vi "run_vi.vi"(6 "wait for reply (T)":bool=TRUE, 8 "error in":errorcluster, 9 "open_frontpanel":bool, 10 "vi_id":i32) -> (0 "error out":errorcluster, 1 "timed out?":bool)   [LabVIEW 2025, in "Scripting Server.lvlib"]
doc: "Runs a VI specified by VI ID and brings the frontpanel to foreground if open_frontpanel is set to True."
uses:
  Scripting Server.lvlib
  Run VI Argument--cluster.ctl
  Run VI (Reply Payload)--cluster.ctl
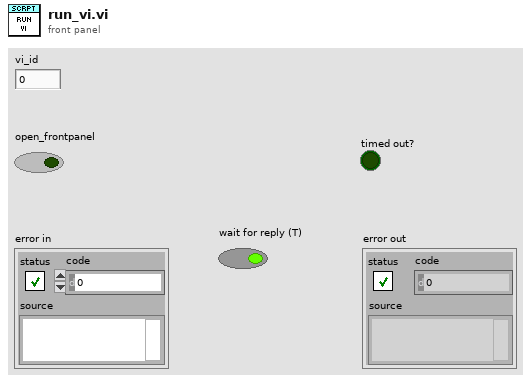
[diagram p1: front panel]
types:
  T1 = typedef "Scripting Server.lvlib/Run VI Argument--cluster.ctl" = cluster{"VI ID":i32, "open_frontpanel":bool, "Wait Notifier":refnum<notifier>, "wait for reply":bool}
  T2 = typedef "Scripting Server.lvlib/Request Events--cluster.ctl" = cluster{"Stop Module":refnum<user-event>, "Show Panel":refnum<user-event>, "Hide Panel":refnum<user-event>, "Get Module Execution Status":refnum<user-event>, "Show Diagram":refnum<user-event>, "New VI":refnum<user-event>, "Add Object":refnum<user-event>, "Connect Objects":refnum<user-event>, "Get Object Terminals":refnum<user-event>, "get vi error list":refnum<user-event>, "Cleanup VI":refnum<user-event>, "create_control":refnum<user-event>, "Run VI":refnum<user-event>}
  T3 = typedef "Scripting Server.lvlib/Run VI (Reply Payload)--cluster.ctl" = cluster{"error":errorcluster}
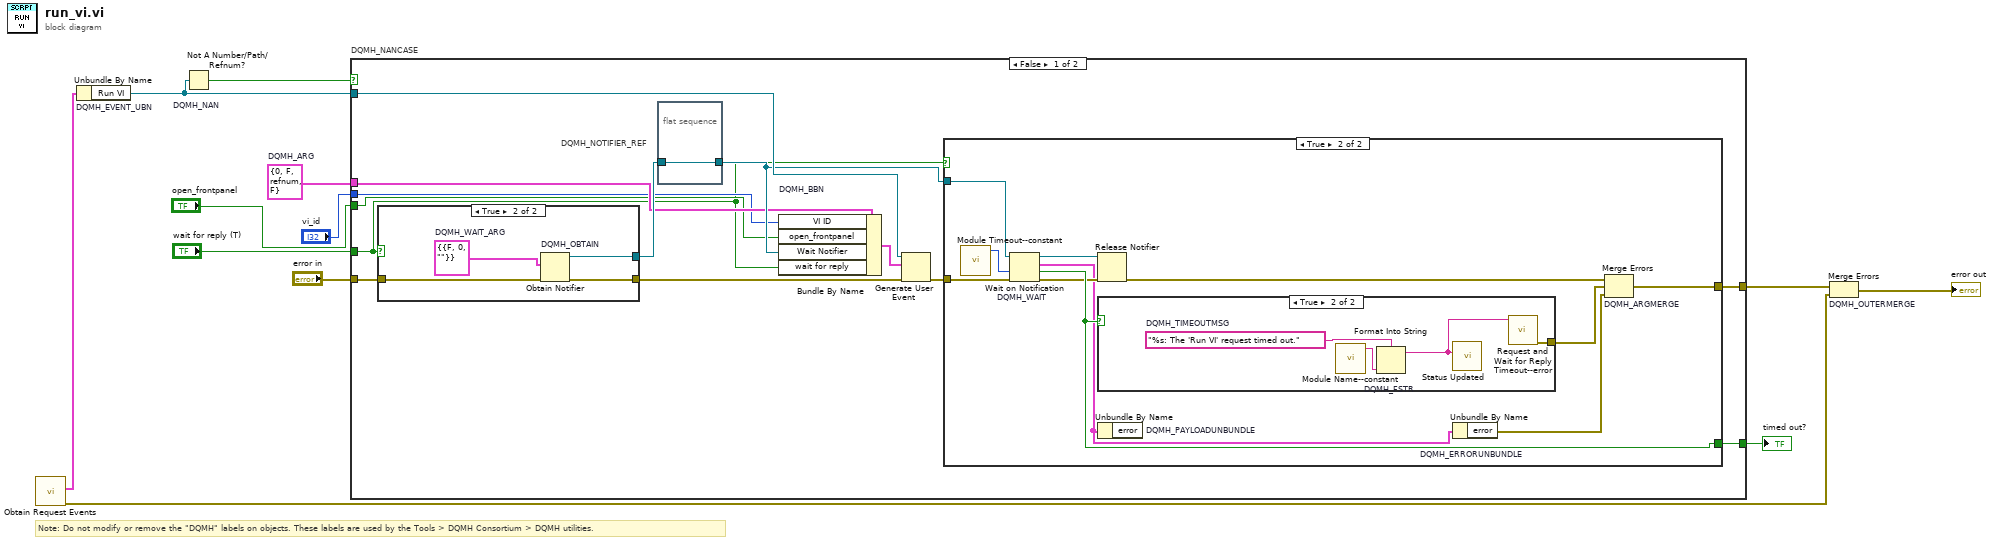
[diagram p0: block diagram]
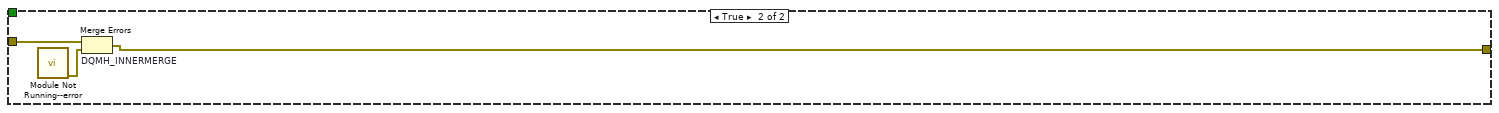
[diagram p5: hidden frame]
diagram:
  w6 = T1 {"VI ID"=0, "open_frontpanel"=FALSE, "Wait Notifier"=refnum, "wait for reply"=FALSE}  # DQMH_ARG
  # "Note: Do not modify or remove the \"DQMH\" labels on objects. These labels are used by the Tools > DQMH Consortium > DQMH utilities."
  n1 = call "Obtain Request Events.vi"() -> ("error out"=w2:errorcluster, "Scripting Server Request Events"=w1:T2)  [unwired: 10 in]
  n2 = Unbundle By Name "DQMH_EVENT_UBN"(w1) -> ("Run VI"=w10:refnum<user-event>)
  n3 = Not A Number/Path/Refnum? "DQMH_NAN"(number/path/refnum=w10) -> (NaN/Path/Refnum?=w9:bool)
  n4 = case "DQMH_NANCASE" shown="False" w9 {
    tunnel: "error in" -> [w25 w50]
    tunnel: w10 -> [w23 _]
    tunnel: [w20 w49] -> w7
    tunnel: [w21 _] -> w8
    tunnel: w6 -> [w16 _]
    tunnel: "vi_id" -> [w15 _]
    tunnel: "open_frontpanel" -> [w14 _]
    tunnel: "wait for reply (T)" -> [w13 _]
    frame False {
      n5 = case shown="True" w13 {
        tunnel: w25 -> [w43 w47]
        tunnel: [w43 w46] -> w22
        tunnel: [_ w44] -> w18
        frame False {
        }
        frame True {
          w45 = T3 {"error"={"status"=FALSE, "code"=0, "source"=""}}  # DQMH_WAIT_ARG
          n6 = Obtain Notifier "DQMH_OBTAIN"(notification data type=w45, error in (no error)=w47) -> (notifier out=w44:refnum<notifier>, error out=w46:errorcluster)  [unwired: 2 in, 1 out]
        }
      }
      n7 = flat-sequence "DQMH_NOTIFIER_REF" {
        tunnel: w18 -> [w26]
        tunnel: [w26] -> w17
        frame #0 {
        }
      }
      n8 = Bundle By Name "DQMH_BBN"(cluster=w16, "VI ID"=w15, "open_frontpanel"=w14, "Wait Notifier"=w17, "wait for reply"=w13) -> (w19:T1)
      n9 = Generate User Event(user event=w23, event data cluster=w19, error in=w22) -> (error out=w24:errorcluster)  [unwired: 1 in, 1 out]
      n10 = case shown="True" w13 {
        tunnel: w24 -> [w27 w38]
        tunnel: w17 -> [_ w37]
        tunnel: [_ w35] -> w21
        tunnel: [w27 w34] -> w20
        frame False {
        }
        frame True {
          n11 = call "Module Timeout--constant.vi"() -> ("Module Timeout"=w28:i32)  [unwired: 11 in]
          n12 = Wait on Notification "DQMH_WAIT"(notifier=w37, timeout in ms (-1)=w28, error in (no error)=w38) -> (notifier out=w36:refnum<notifier>, notification=w29:T3, timed out?=w35:bool, error out=w33:errorcluster)  [unwired: 1 in]
          n13 = Release Notifier(notifier=w36, error in (no error)=w33) -> (error out=w32:errorcluster)  [unwired: 1 in, 2 out]
          n14 = case shown="True" w35 {
            tunnel: [_ w40] -> w30
            frame False {
            }
            frame True {
              w42 = "%s: The 'Run VI' request timed out."  # DQMH_TIMEOUTMSG
              n15 = call "Module Name--constant.vi"() -> ("Module Name"=w39:string)  [unwired: 11 in]
              n16 = Format Into String "DQMH_FSTR"(format string=w42, w39) -> (resulting string=w41:string)  [unwired: 2 in, 1 out]
              n17 = call "Status Updated.vi"("Status"=w41) -> ()  [unwired: 10 in, 1 out]
              n18 = call "Request and Wait for Reply Timeout--error.vi"("Error Message"=w41) -> ("error out"=w40:errorcluster)  [unwired: 10 in]
            }
          }
          n19 = Unbundle By Name "DQMH_PAYLOADUNBUNDLE"(w29) -> ()  [unwired: 1 out]
          n20 = Unbundle By Name "DQMH_ERRORUNBUNDLE"(w29) -> ("error"=w31:errorcluster)
          n21 = Merge Errors "DQMH_ARGMERGE"(w32, w30, w31) -> (w34:errorcluster)
        }
      }
    }
    frame True {
      n22 = call "Module Not Running--error.vi"() -> ("error out"=w48:errorcluster)  [unwired: 11 in]
      n23 = Merge Errors "DQMH_INNERMERGE"(w50, w48) -> (w49:errorcluster)
    }
  }
  "timed out?" <- w8
  n24 = Merge Errors "DQMH_OUTERMERGE"(w7, w2) -> (→"error out":errorcluster)
